vi "ShowFrontPanelHelper.vi"(10 "Data":T1, 11 "VI in":refnum<vi>) -> (0 "error out":errorcluster)   [LabVIEW 2024, in "Module.lvclass"]
uses:
  Module.lvclass
  Module.lvclass/Module.ctl
  Show Front Panel--Args.ctl
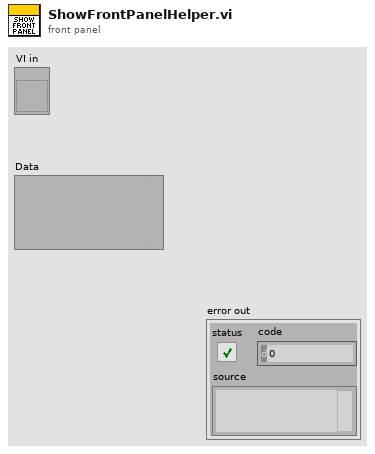
[diagram p1: front panel]
types:
  T1 = typedef "Module.lvclass/Show Front Panel--Args.ctl" = variant
  T2 = enum32{"Invalid", "Standard", "Closed", "Hidden", "Minimized", "Maximized"}
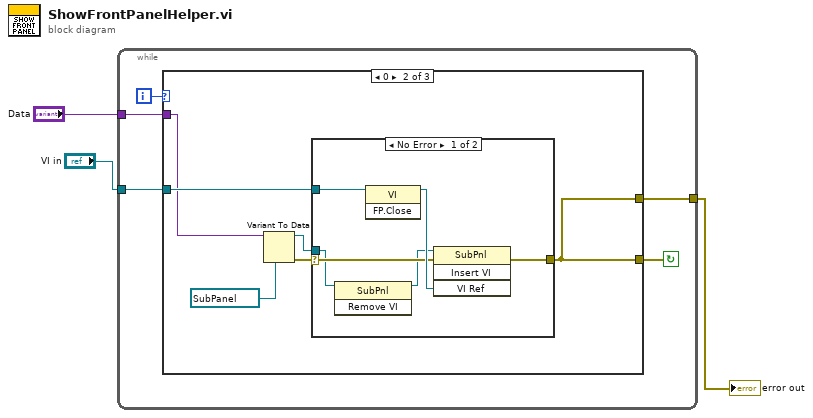
[diagram p0: block diagram]
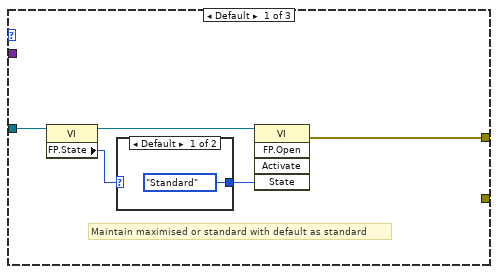
[diagram p2: hidden frame]
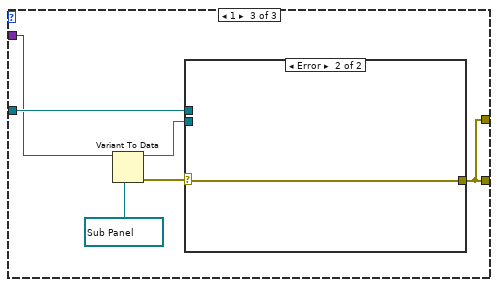
[diagram p5: hidden frame]
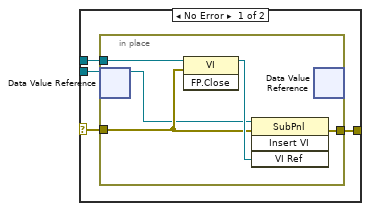
[diagram p6: hidden frame]
diagram:
  n1 = while {
    tunnel: "VI in" -> [w7]
    tunnel: [w5] -> w3
    tunnel: "Data" -> [w4]
    i -> [w8]
    stop <- w6 continue-if-true
    n2 = case shown="0" w8 {
      tunnel: w7 -> [w13 w21 w34]
      tunnel: [_ w20 w33] -> w6
      tunnel: w4 -> [_ w17 w32]
      tunnel: [w12 w20 w33] -> w5
      frame Default {
        # "Maintain maximised or standard with default as standard"
        n3 = property class="VI"(reference=w13) -> (reference out=w11:refnum<vi>, "FP.State"=w10:T2)  [unwired: 1 in, 1 out]
        n4 = case shown="Default" w10 {
          selector: w10 -> [_ w15]
          tunnel: [T2."Standard" ("FP.State") w15] -> w9
          frame Default {
          }
          frame "Standard", "Maximized" {
          }
        }
        n5 = invoke class="VI" method="FP.Open"(reference=w11, "State"=w9) -> (error out=w12:errorcluster)  [unwired: 3 in, 4 out]
      }
      frame 0 {
        n6 = Variant To Data(type=refnum<vi> refnum ("Sub Panel"), Variant=w17) -> (data=w18:refnum<vi>, error out=w19:errorcluster)  [unwired: 1 in]
        n7 = case shown="No Error" w19 {
          selector: w19 -> [w24 w28]
          tunnel: w18 -> [w22 _]
          tunnel: w21 -> [w27 _]
          tunnel: [w25 w28] -> w20
          frame No Error {
            n8 = invoke class="SubPnl" method="Remove VI"(reference=w22) -> (reference out=w23:refnum<vi>)  [unwired: 2 in, 2 out]
            n9 = invoke class="VI" method="FP.Close"(reference=w27) -> (reference out=w26:refnum<vi>)  [unwired: 2 in, 2 out]
            n10 = invoke class="SubPnl" method="Insert VI"(reference=w23, error in=w24, "VI Ref"=w26) -> (error out=w25:errorcluster)  [unwired: 1 in, 3 out]
          }
          frame Error {
          }
        }
      }
      frame 1 {
        n11 = Variant To Data(type=refnum<data-value> refnum ("data value reference"), Variant=w32) -> (data=w29:refnum<data-value>, error out=w30:errorcluster)  [unwired: 1 in]
        n12 = case shown="Error" w30 {
          selector: w30 -> [w36 w44]
          tunnel: w34 -> [w38 _]
          tunnel: [w37 w44] -> w33
          tunnel: w29 -> [w35 _]
          frame No Error {
            n13 = in-place {
              in-place-border: w38 -> [w43]
              in-place-border: [w41] -> w37
              in-place-border: w36 -> [w40]
              n14 = in-place-dvr #1(w35) -> (w39:refnum<vi>)  [unwired: 1 out]
              n15 = invoke class="VI" method="FP.Close"(reference=w43, error in=w40) -> (reference out=w42:refnum<vi>)  [unwired: 1 in, 2 out]
              n16 = invoke class="SubPnl" method="Insert VI"(reference=w39, error in=w40, "VI Ref"=w42) -> (error out=w41:errorcluster)  [unwired: 1 in, 3 out]
              n17 = in-place-dvr #1() -> ()  [unwired: 1 in, 2 out]
            }
          }
          frame Error {
          }
        }
      }
    }
  }
  "error out" <- w3
